vi "mqttCmdPublishCompleteCommand.vi"(9 "messageID":u16, 11 "error in (no error)":errorcluster) -> (15 "error out":errorcluster)   [LabVIEW 2019]
uses:
  mqttTypedef/mqttMessageType.ctl
  mqttTypedef/mqttQOSlevel.ctl
  mqttCmd.lvclass
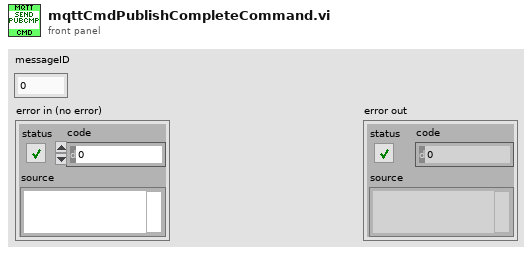
[diagram p1: front panel]
types:
  T1 = typedef "mqttQOSlevel.ctl" = enum8{"At most once", "At least once", "Exactly once", "Reserved"}
  T2 = typedef "mqttMessageType.ctl" = enum32{"Reserved", "CONNECT", "CONNACK", "PUBLISH", "PUBACK", "PUBREC", "PUBREL", "PUBCOMP", "SUBSCRIBE", "SUBACK", "UNSUBSCRIBE", "UNSUBACK", "PINGREQ", "PINGRESP", "DISCONNECT", "Reserved2"}
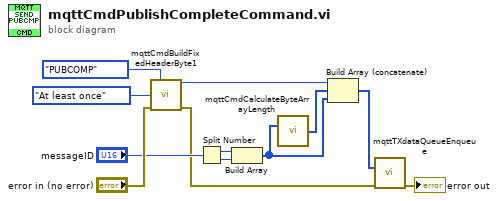
[diagram p0: block diagram]
diagram:
  n1 = call "mqttCmdBuildFixedHeaderByte1.vi"("MessageType"=mqttMessageType."PUBCOMP", "QoS (At most once)"=mqttQOSlevel."At least once", "error in (no error)"="error in (no error)") -> ("byte1"=w1:u8, "error out"=w4:errorcluster)  [unwired: 11 in]
  n2 = Split Number(x="messageID") -> (hi(x)=w8:u8, lo(x)=w7:u8)
  n3 = Build Array(w8, w7) -> (w9:u8[])
  n4 = call "mqttCmdCalculateByteArrayLength.vi"("byteArry in"=w9) -> ("length out"=w6:u8[])  [unwired: 13 in, 1 out]
  n5 = Build Array (concatenate)(w1, w6, w9) -> (w2:u8[])
  n6 = call "mqttTXdataQueueEnqueue.vi"("data in"=w2, "error in (no error)"=w4) -> ("error out"=→"error out":errorcluster)  [unwired: 13 in]
